vi "write offsets.vi"(8 "error in (no error)":errorcluster, 9 "Offset Value":dbl[](array[numeric]), 10 "Offset IOName":string[](array[string]), 11 "offsets.ini file":path) -> (0 "error out":errorcluster, 2 "offsets":T1)   [LabVIEW 2017, in "DAQ.lvclass"]
doc: "Developed by Kevin Thompson\nkevin@thompsonengineering.net\n\nCopyright 2018-2020\nThompson Engineering, LLC"
uses:
  DAQ.lvclass
  DataTypes/offsets cluster.ctl
  <vilib>/Utility/config.llb/NI_LVConfig.lvlib
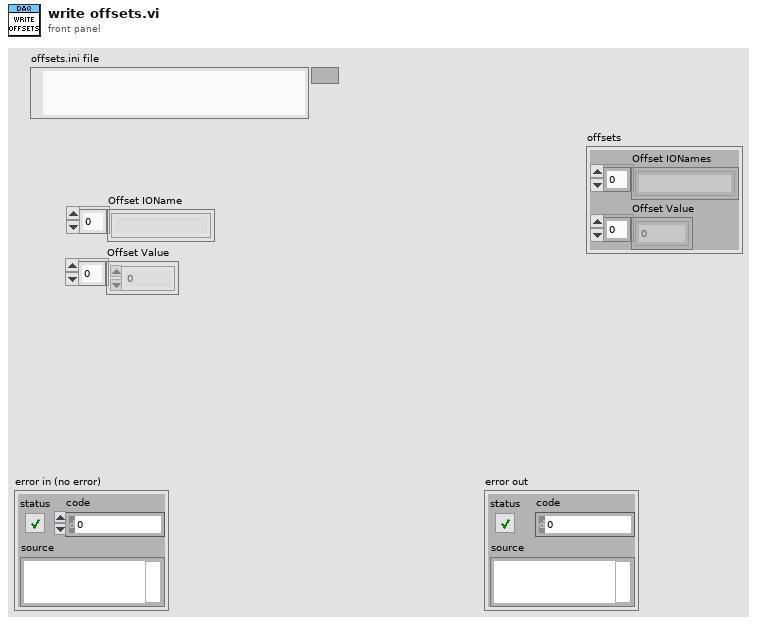
[diagram p1: front panel]
types:
  T1 = typedef "DAQ.lvclass/offsets cluster.ctl" = cluster{"Offset IONames":string[], "Offset Value":dbl[]}
  T2 = typedef "NI_LVConfig.lvlib/Config Data RefNum.ctl" = refnum<k1>
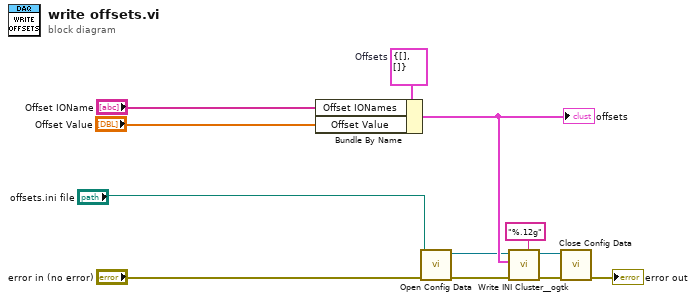
[diagram p0: block diagram]
diagram:
  w11 = T1 {"Offset IONames"=[], "Offset Value"=[]}  # Offsets
  n1 = Bundle By Name(cluster=w11, "Offset IONames"="Offset IOName", "Offset Value"="Offset Value") -> (w12:T1)
  "offsets" <- w12
  n2 = call <vilib>:"Open Config Data.vi"("error in (no error)"="error in (no error)", "configuration file path"="offsets.ini file") -> ("error out"=w8:errorcluster, "refnum"=w5:T2)  [unwired: 7 in, 1 out]
  n3 = call <userlib>:"Write INI Cluster__ogtk.vi"("float number format (optional)"="%.12g", "error in (no error)"=w8, "INI Fomatted Cluster"=w12, "refnum"=w5) -> ("error out"=w7:errorcluster, "dup refnum"=w6:T2)  [unwired: 6 in]
  n4 = call <vilib>:"Close Config Data.vi"("error in (no error)"=w7, "refnum"=w6) -> ("error out"=→"error out":errorcluster)  [unwired: 8 in, 1 out]
